vi "RealAmountOfGPCSamples.vi"(1 "GPC Interval":dbl, 2 "tres2":dbl) -> (0 "Real amount of samples":dbl)   [LabVIEW 2018]
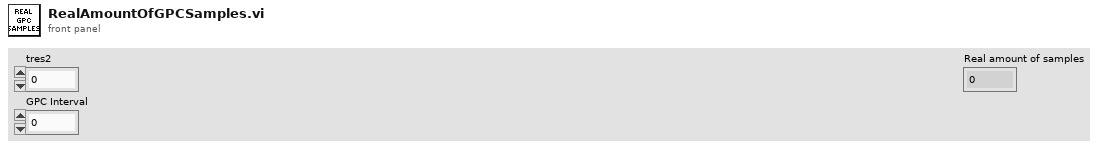
[diagram p1: front panel]
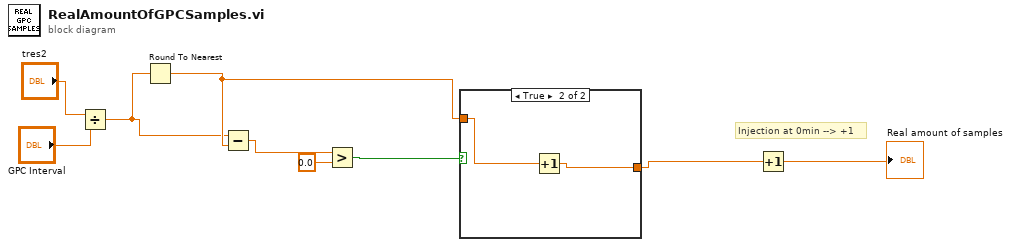
[diagram p0: block diagram]
diagram:
  # "Injection at 0min --> +1"
  n1 = Divide(x="tres2", y="GPC Interval") -> (x/y=w3:dbl)
  n2 = Round To Nearest(number=w3) -> (nearest integer value=w6:dbl)
  n3 = Subtract(x=w3, y=w6) -> (x-y=w9:dbl)
  n4 = Greater?(x=w9, y=0.0) -> (0:w7:bool)
  n5 = case shown="True" w7 {
    tunnel: [w10 w12] -> w2
    tunnel: w6 -> [w10 w11]
    frame False {
    }
    frame True {
      n6 = Increment(x=w11) -> (x+1=w12:dbl)
    }
  }
  n7 = Increment(x=w2) -> (x+1=→"Real amount of samples":dbl)
